vi "Compute Min Image.vi"(8 "error in (no error)":errorcluster, 10 "New Image":T1, 11 "Min Image Dst":T1) -> (0 "error out":errorcluster, 3 "Min Image":T1)   [LabVIEW 2021, in "Image.lvlib"]
uses:
  <vilib>/vision/Image Controls.llb/IMAQ Image.ctl
  Image.lvlib
  <vilib>/vision/NI_Vision_Development_Module.lvlib
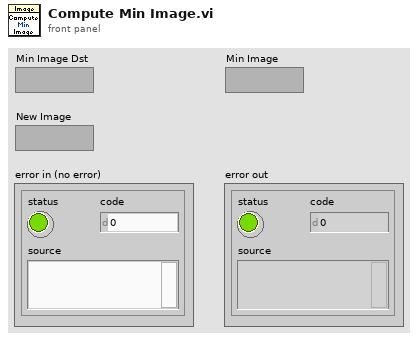
[diagram p1: front panel]
types:
  T1 = typedef "IMAQ Image.ctl" = refnum<image>
  T2 = typedef "Image Type" = u32
  T3 = enum32{"Average", "Min", "Max", "Clear  if < ", "Clear  if < or =", "Clear  if =", "Clear  if > or =", "Clear  if >"}
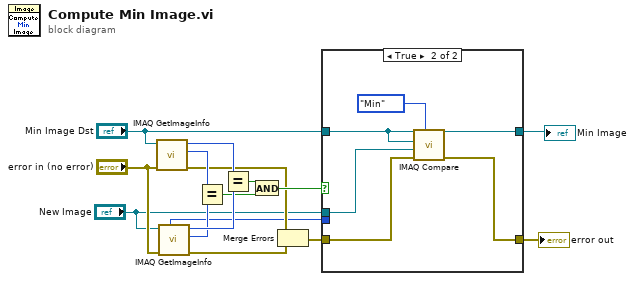
[diagram p0: block diagram]
diagram:
  n1 = call "IMAQ GetImageInfo"("error in (no error)"="error in (no error)", "Image"="Min Image Dst") -> ("error out"=w7:errorcluster, "Y Resolution"=w13:i32, "X Resolution"=w15:i32)  [unwired: 2 in, 5 out]
  n2 = call "IMAQ GetImageInfo"("error in (no error)"="error in (no error)", "Image"="New Image") -> ("error out"=w8:errorcluster, "Y Resolution"=w12:i32, "X Resolution"=w14:i32, "Image Type"=w4:T2)  [unwired: 2 in, 4 out]
  n3 = Equal?(x=w13, y=w12) -> (x = y?=w10:bool)
  n4 = Equal?(x=w15, y=w14) -> (x = y?=w11:bool)
  n5 = And(x=w11, y=w10) -> (x .and. y?=w9:bool)
  n6 = Merge Errors(w7, w8) -> (w6:errorcluster)
  n7 = case shown="True" w9 {
    tunnel: "Min Image Dst" -> [w17 w21]
    tunnel: w6 -> [w18 w23]
    tunnel: [w18 w22] -> w5
    tunnel: w4 -> [_ _]
    tunnel: "New Image" -> [_ w24]
    tunnel: [w17 w20] -> w1
    frame False {
      # "Not the same image dimensions"
    }
    frame True {
      n8 = call "IMAQ Compare"("Operator"=T3."Min", "error in (no error)"=w23, "Image Src B"=w24, "Image Dst"=w21, "Image Src A"=w21) -> ("error out"=w22:errorcluster, "Image Dst Out"=w20:T1)  [unwired: 5 in]
    }
  }
  "error out" <- w5
  "Min Image" <- w1
